vi "Configure Reference Oscillator.vi"(8 "error in (no error)":errorcluster, 10 "Reference Oscillator (Internal)":enum16{"Internal", "External"}(ring), 11 "MXA in":refnum<class "MXA.lvclass">) -> (0 "error out":errorcluster, 3 "MXA out":refnum<class "MXA.lvclass">)   [LabVIEW 2020, in "MXA.lvclass"]
uses:
  MXA.lvclass
  C:/Sandbox/Git_Sandbox/WiSpry Test Framework source code (LV20)/WiSpry Test Framework/Instruments/Instrument.lvclass
  Instrument.lvclass/Instrument.ctl
  Instrument.lvclass
  <instrlib>/Agilent MXA Series/Agilent MXA Series.lvlib
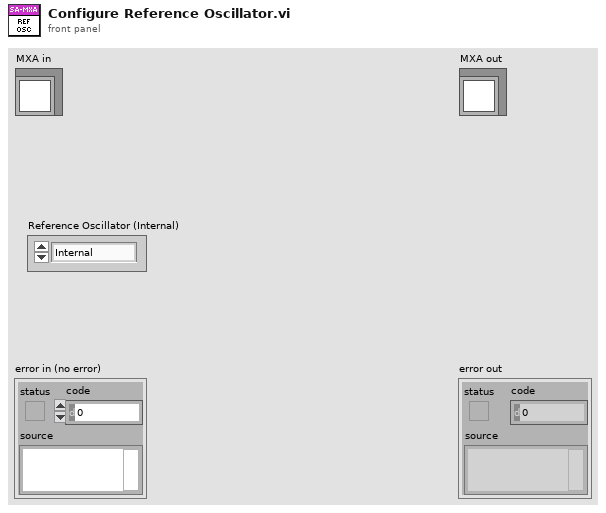
[diagram p1: front panel]
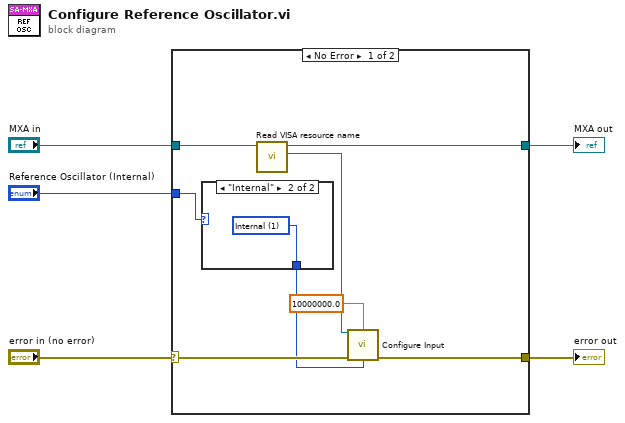
[diagram p0: block diagram]
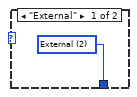
[diagram p2: hidden frame]
diagram:
  n1 = case shown="No Error" "error in (no error)" {
    selector: "error in (no error)" -> [w10 w17]
    tunnel: "MXA in" -> [w13 w16]
    tunnel: [w9 w17] -> w5
    tunnel: [w12 w16] -> w4
    tunnel: "Reference Oscillator (Internal)" -> [w7 _]
    frame No Error {
      n2 = case shown="\"Internal\"" w7 {
        tunnel: [w14 w15] -> w8
        frame "External" {
          w14 = 2 items=["Sense", "Internal", "External"] ("Frequency Reference In  (0:Sense)")
        }
        frame "Internal" {
          w15 = 1 items=["Sense", "Internal", "External"] ("Frequency Reference In  (0:Sense)")
        }
      }
      n3 = call "Read VISA resource name.vi"("Instrument in"=w13) -> ("VISA resource name"=w11:refnum<visa-resource-name>, "Instrument out"=w12:refnum<class "MXA.lvclass">)  [unwired: 9 in]
      n4 = call <instrlib>:"Configure Input.vi"("VISA resource name"=w11, "External Frequency (0 Hz)"=10000000.0, "error in (no error)"=w10, "Frequency Reference In  (0:Sense)"=w8) -> ("error out"=w9:errorcluster)  [unwired: 10 in, 1 out]
    }
    frame Error {
    }
  }
  "error out" <- w5
  "MXA out" <- w4
